vi "CreateCloseEvent.vi"(8 "error in (no error)":errorcluster, 11 "Menu in":refnum<class "VIActivation.lvclass">) -> (0 "error out":errorcluster, 2 "ExitEvent":refnum<user-event>, 3 "Menu out":refnum<class "VIActivation.lvclass">)   [LabVIEW 2021, in "VIActivation.lvlib" / "VIActivation.lvclass"]
uses:
  VIActivation.lvclass
  GetCloseEventRef.vi
  SetCloseEventRef.vi
  VIActivation.lvclass/VIActivation.ctl
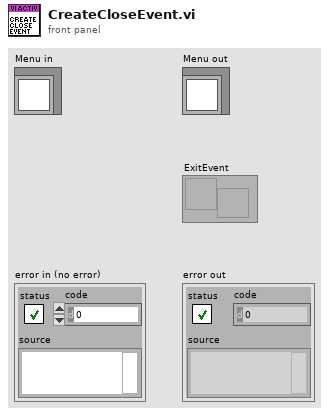
[diagram p1: front panel]
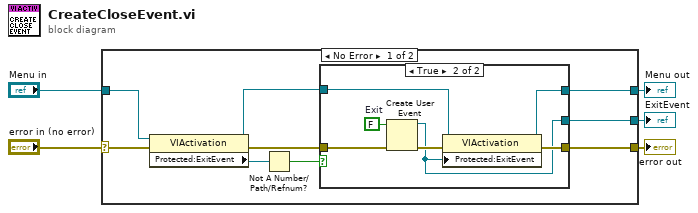
[diagram p0: block diagram]
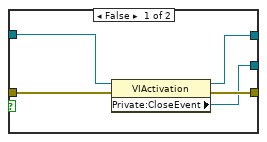
[diagram p2: hidden frame]
diagram:
  n1 = case shown="No Error" "error in (no error)" {
    selector: "error in (no error)" -> [w10 w28]
    tunnel: [w8 w28] -> w4
    tunnel: [w14 w27] -> w2
    tunnel: "Menu in" -> [w12 w27]
    tunnel: [w6 _] -> w1
    frame No Error {
      n2 = property class="VIActivation"(reference=w12, error in=w10) -> (reference out=w11:refnum<class "VIActivation.lvclass">, error out=w9:errorcluster, "Protected:ExitEvent"=w7:refnum<user-event>)
      n3 = Not A Number/Path/Refnum?(number/path/refnum=w7) -> (NaN/Path/Refnum?=w13:bool)
      n4 = case shown="True" w13 {
        tunnel: w11 -> [w18 w26]
        tunnel: [w19 w25] -> w14
        tunnel: [w17 w24] -> w8
        tunnel: w9 -> [w15 w23]
        tunnel: [w16 w21] -> w6
        frame False {
          n5 = property class="VIActivation"(reference=w18, error in=w15) -> (reference out=w19:refnum<class "VIActivation.lvclass">, error out=w17:errorcluster, "Private:CloseEvent"=w16:refnum<user-event>)
        }
        frame True {
          w20 = FALSE  # Exit
          n6 = Create User Event(user event datatype=w20, error in=w23) -> (user event=w21:refnum<user-event>, error out=w22:errorcluster)
          n7 = property class="VIActivation"(reference=w26, error in=w22, "Protected:ExitEvent"=w21) -> (reference out=w25:refnum<class "VIActivation.lvclass">, error out=w24:errorcluster)
        }
      }
    }
    frame Error {
    }
  }
  "error out" <- w4
  "Menu out" <- w2
  "ExitEvent" <- w1
